vi "readSamples.vi"(8 "error in (no error)":errorcluster, 10 "NI9870 in":refnum<class "NI9870.lvclass">, 11 "RTDisplacement in":refnum<class "RTDisplacement.lvclass">) -> (0 "error out":errorcluster, 1 "Samples":T1[](array[typedef]), 2 "NI9870 out":refnum<class "NI9870.lvclass">, 3 "RTDisplacement out":refnum<class "RTDisplacement.lvclass">)   [LabVIEW 2016, in "RTDisplacement.lvlib" / "RTDisplacement.lvclass"]
uses:
  RTDisplacement.lvclass
  Scratch/RTNI9870/NI9871/NI9870.lvclass
  DataTypes/DisplacementData.ctl
  RTDisplacement.lvlib
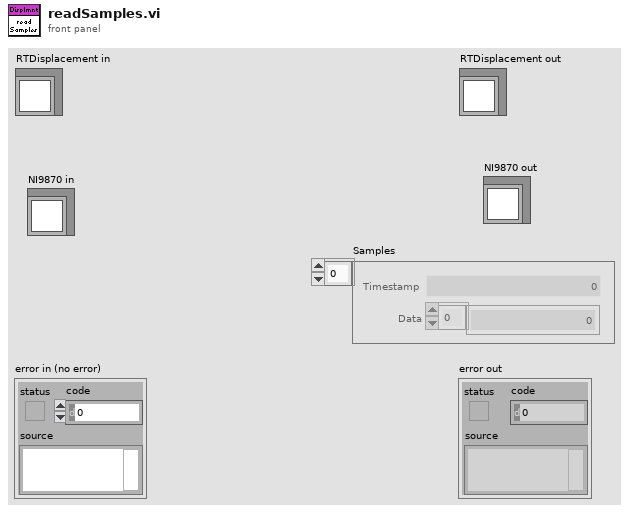
[diagram p1: front panel]
types:
  T1 = typedef "RTDisplacement.lvlib/DisplacementData.ctl" = cluster{"Timestamp":u64, "Data":dbl[]}
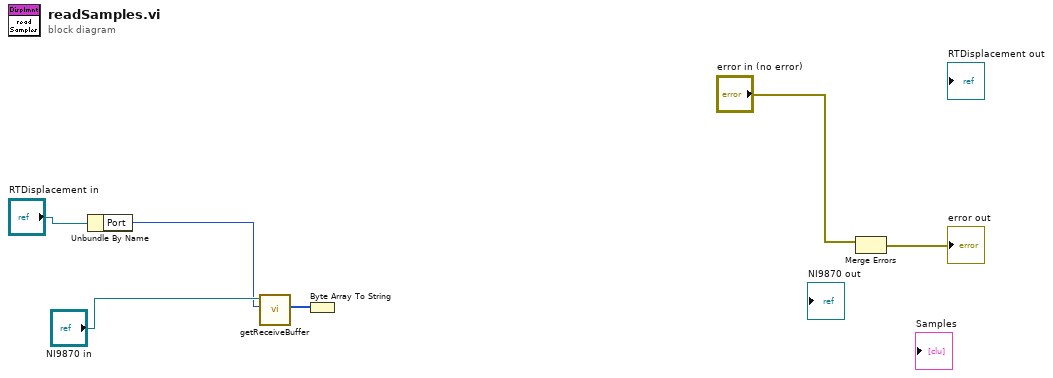
[diagram p0: block diagram]
diagram:
  n1 = Unbundle By Name("RTDisplacement in") -> ("Port"=w2:u8)
  n2 = call "getReceiveBuffer.vi"("Port"=w2, "NI9870 in"="NI9870 in") -> ("Buffer"=w1:u8[])  [unwired: 7 in, 2 out]
  n3 = Byte Array To String(unsigned byte array=w1) -> ()  [unwired: 1 out]
  n4 = Merge Errors("error in (no error)") -> (→"error out":errorcluster)  [unwired: 1 in]
